vi "Main.vi"(11 "Module Admin":refnum<class "Delacor_lib_QMH_Module Admin.lvclass">) -> ()   [LabVIEW 2020, in "Acquisition.lvlib"]
doc: "This template is based off of the Queued Message Handler design pattern and the Queued Message Handler project template that ships with LabVIEW.\n\nThe main difference is that the queue is private to this module and communication between modules is performed via Broadcast and Request events.\n\nRequest events are wrapped in public API methods and are handled in the Event Handling Loop (EHL) of this VI. Any module can register for Broadcast events sent by this module. The EHL generates messages based on user interface actions.\n\nThe Message Handling Loop (MHL) processes messages generated by the EHL, or by other messages. The messages are string values, so new messages can be added easily to the Message Cases case structure in the MHL. Each message cluster can also provide an optional value for Message Data, which is a variant that can be converted to whatever message-specific data is required.\n_____\nBased on Delacor QMH Project Template 4.0.0.47.\n_____\nBased on DQMH Project Template 6.0.0.91."
uses:
  Acquisition.lvlib
  <vilib>/Delacor/Delacor QMH/Libraries/Module Admin_class/Delacor_lib_QMH_Module Admin.lvclass
  Module Data--cluster.ctl
  Settings Editor/DAQmx Timing--cluster.ctl
  Settings Editor/DAQmx Trigger Settings--cluster.ctl
  Settings Editor/DAQmx Config--cluster.ctl
  Stop Argument--cluster.ctl
  <vilib>/Delacor/Delacor QMH/Libraries/Message Queue_class/Delacor_lib_QMH_Message Queue.lvclass/Delacor_lib_QMH_Message Queue.ctl
  <vilib>/Delacor/Delacor QMH/Libraries/Module Admin_class/Delacor_lib_QMH_Module Admin.lvclass/Delacor_lib_QMH_Module Admin.ctl
  Start Acquiring Argument--cluster.ctl
  Start Acquiring (Reply Payload)--cluster.ctl
  Stop Acquiring Argument--cluster.ctl
  Settings Editor/Update Application Settings (Reply Payload)--cluster.ctl
  Settings Editor/Settings--cluster.ctl
  <vilib>/Utility/miscctls.llb/LVPointTypeDef.ctl
  <vilib>/Delacor/Delacor QMH/Libraries/Message Queue_class/Delacor_lib_QMH_Enqueue Message (Single).vi
  <vilib>/Delacor/Delacor QMH/Libraries/Module Admin_class/Delacor_lib_QMH_Get External Launch.vi
  <vilib>/Utility/error.llb/Error Cluster From Error Code.vi
  <vilib>/ErrorRing/Error Ring.xnode
  <vilib>/Delacor/Delacor QMH/Libraries/Message Queue_class/Delacor_lib_QMH_Message Queue.lvclass
  Settings Editor/Settings Editor.lvlib
  Logger/Logger.lvlib
panel:
  out "Settings":T1={"HW Refnum"="", "DAQmx Timing Settings"={"rate"=0.0, "source"="OnboardClock", "sample mode"=10178, "samples per channel"=1000}, "Trigger Settings"={"Trigger Type"=enum."No Trigger", "Digital Start"={"Source"="", "Digital Start Trigger Edge"=10280}, "Digital Pause"={"Source"="", "Digital Pause Trigger Pause When"=10192}, "Digital Reference"={"Source"="", "Digital Start Trigger Edge"=10280, "Digital Reference Pretrigger Samples"=0}, "Analog Start"={"Source"="", "Analog Slope"=10280, "Analog Start Trigger Hysteresis"=0.0, "Analog Start Trigger Level"=0.0}, "Analog Pause"={"Source"="", "Analog Start Trigger Level"=0.0, "Analog Pause Trigger Pause When"=10093}, "Analog Reference"={"Source"="", "Slope"=10280, "Pretrigger Samples"=0, "Level"=0.0}, "Time Start"={"Select Time\nManually"=FALSE, "When"=timestamp(0 s since 1904-01-01)}}, "DAQmx Config"=[], "Calibration Array"=[{"Slope"=1.0, "Offset"=0.0}]} {"DAQmx Config"."Unit" items=["Volts", "From Custom Scale"]; "Trigger Settings"."Time Start"."When" format="%<%x %.3X>T"; "Trigger Settings"."Analog Reference"."Level" format="%0.2f"; "Trigger Settings"."Analog Reference"."Slope" items=["Rising"=10280, "Falling"=10171]; "Trigger Settings"."Analog Pause"."Analog Pause Trigger Pause When" items=["Above Level"=10093, "Below Level"=10107]; "Trigger Settings"."Analog Pause"."Analog Start Trigger Level" format="%0.2f"; "Trigger Settings"."Analog Start"."Analog Start Trigger Level" format="%0.2f"; "Trigger Settings"."Analog Start"."Analog Start Trigger Hysteresis" format="%.2f"; "Trigger Settings"."Analog Start"."Analog Slope" items=["Rising"=10280, "Falling"=10171]; "Trigger Settings"."Digital Reference"."Digital Start Trigger Edge" items=["Rising"=10280, "Falling"=10171]; "Trigger Settings"."Digital Pause"."Digital Pause Trigger Pause When" items=["High"=10192, "Low"=10214]; "Trigger Settings"."Digital Start"."Digital Start Trigger Edge" items=["Rising"=10280, "Falling"=10171]; "DAQmx Timing Settings"."sample mode" items=["Finite Samples"=10178, "Continuous Samples"=10123, "Hardware Timed Single Point"=12522]; "DAQmx Timing Settings"."rate" format="%0.2f"}
  out "Graph Data":waveform(dbl)[](array[waveform])
  out "error out":errorcluster
  # "This is a headless module. Show its panel to confirm that the Settings are updated correctly and other debugging tasks. Use the Settings Editor to change the settings for this module."
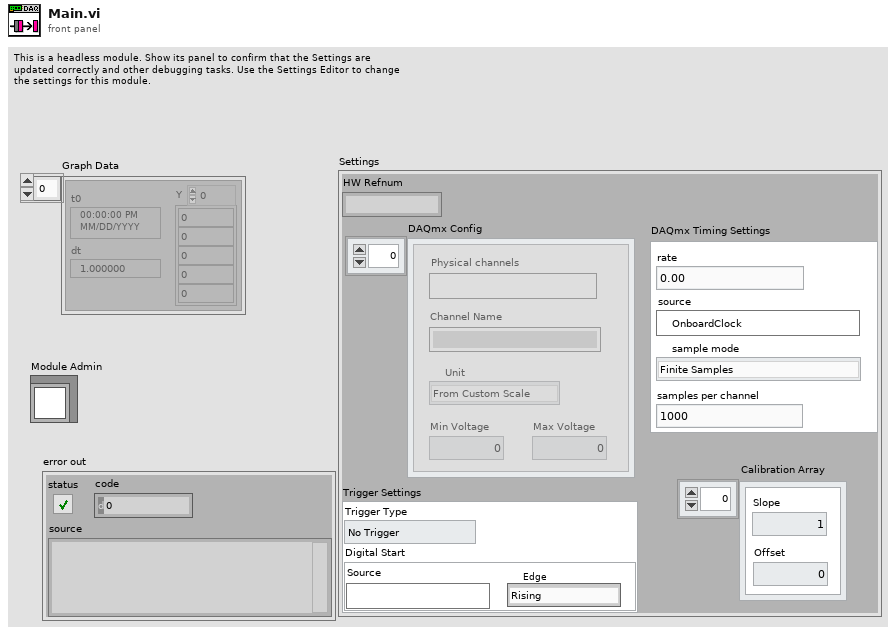
[diagram p1: front panel]
types:
  T1 = typedef "Acquisition.lvlib/Module Data--cluster.ctl" = cluster{"HW Refnum":string, "DAQmx Timing Settings":T2, "Trigger Settings":T3, "DAQmx Config":T4, "Calibration Array":cluster{"Slope":dbl, "Offset":dbl}[]}
  T2 = typedef "Settings Editor.lvlib/DAQmx Timing--cluster.ctl" = cluster{"rate":dbl, "source":tag, "sample mode":i32, "samples per channel":i32}
  T3 = typedef "Settings Editor.lvlib/DAQmx Trigger Settings--cluster.ctl" = cluster{"Trigger Type":enum32{"No Trigger", "Digital Start", "Digital Pause", "Digital Reference", "Analog Start", "Analog Pause", "Analog Reference", "Time Start"}, "Digital Start":cluster{"Source":tag, "Digital Start Trigger Edge":i32}, "Digital Pause":cluster{"Source":tag, "Digital Pause Trigger Pause When":i32}, "Digital Reference":cluster{"Source":tag, "Digital Start Trigger Edge":i32, "Digital Reference Pretrigger Samples":u32}, "Analog Start":cluster{"Source":string, "Analog Slope":i32, "Analog Start Trigger Hysteresis":dbl, "Analog Start Trigger Level":dbl}, "Analog Pause":cluster{"Source":string, "Analog Start Trigger Level":dbl, "Analog Pause Trigger Pause When":i32}, "Analog Reference":cluster{"Source":string, "Slope":i32, "Pretrigger Samples":u32, "Level":dbl}, "Time Start":cluster{"Select Time\nManually":bool, "When":timestamp}}
  T4 = typedef "Settings Editor.lvlib/DAQmx Config--cluster.ctl" = cluster{"Physical channels":tag, "Channel Name":string, "Unit":i32, "Min Voltage":dbl, "Max Voltage":dbl}[]
  T5 = typedef "Settings Editor.lvlib/Broadcast Events--cluster.ctl" = cluster{"Module Did Init":refnum<user-event>, "Status Updated":refnum<user-event>, "Error Reported":refnum<user-event>, "Module Did Stop":refnum<user-event>, "Update Module Execution Status":refnum<user-event>, "Application Settings Updated":refnum<user-event>}
  T6 = typedef "Acquisition.lvlib/Request Events--cluster.ctl" = cluster{"Stop Module":refnum<user-event>, "Show Panel":refnum<user-event>, "Hide Panel":refnum<user-event>, "Get Module Execution Status":refnum<user-event>, "Show Diagram":refnum<user-event>, "Stop Acquiring":refnum<user-event>, "Wakeup Helper Loop":refnum<user-event>, "Change Settings":refnum<user-event>, "Calibrate DAQ":refnum<user-event>, "Start Acquiring":refnum<user-event>}
  T7 = enum32{"invalid lock state", "Not Locked", "Locked (No Password)", "Password-protected"}
  T8 = typedef "Acquisition.lvlib/Stop Argument--cluster.ctl" = cluster{"Origin":string, "Exit via Stop Module Req?":bool, "Wait for Module to stop?":bool}
  T9 = typedef "Acquisition.lvlib/Start Acquiring Argument--cluster.ctl" = cluster{"Wait Notifier":refnum<notifier>, "wait for reply":bool}
  T10 = typedef "Acquisition.lvlib/Stop Acquiring Argument--cluster.ctl" = cluster{"Boolean":bool}
  T11 = typedef "Settings Editor.lvlib/Update Application Settings (Reply Payload)--cluster.ctl" = cluster{"Settings":T12, "Update Settings_error":errorcluster}
  T12 = typedef "Settings Editor.lvlib/Settings--cluster.ctl" = cluster{"Calibration Array":cluster{"Slope":dbl, "Offset":dbl}[], "Hardware Config Cluster":T4, "Trigger Settings":T3, "Log File Base Path":path, "DAQmx Timing Settings":T2}
  T13 = typedef "LVPointTypeDef.ctl" = cluster{"Horizontal":i16, "Vertical":i16}
  T14 = enum32{"Invalid", "Standard", "Closed", "Hidden", "Minimized", "Maximized"}
  T15 = typedef "Acquisition.lvlib/Start Acquiring (Reply Payload)--cluster.ctl" = cluster{"HW ID":string, "Start Acquiring_error":errorcluster}
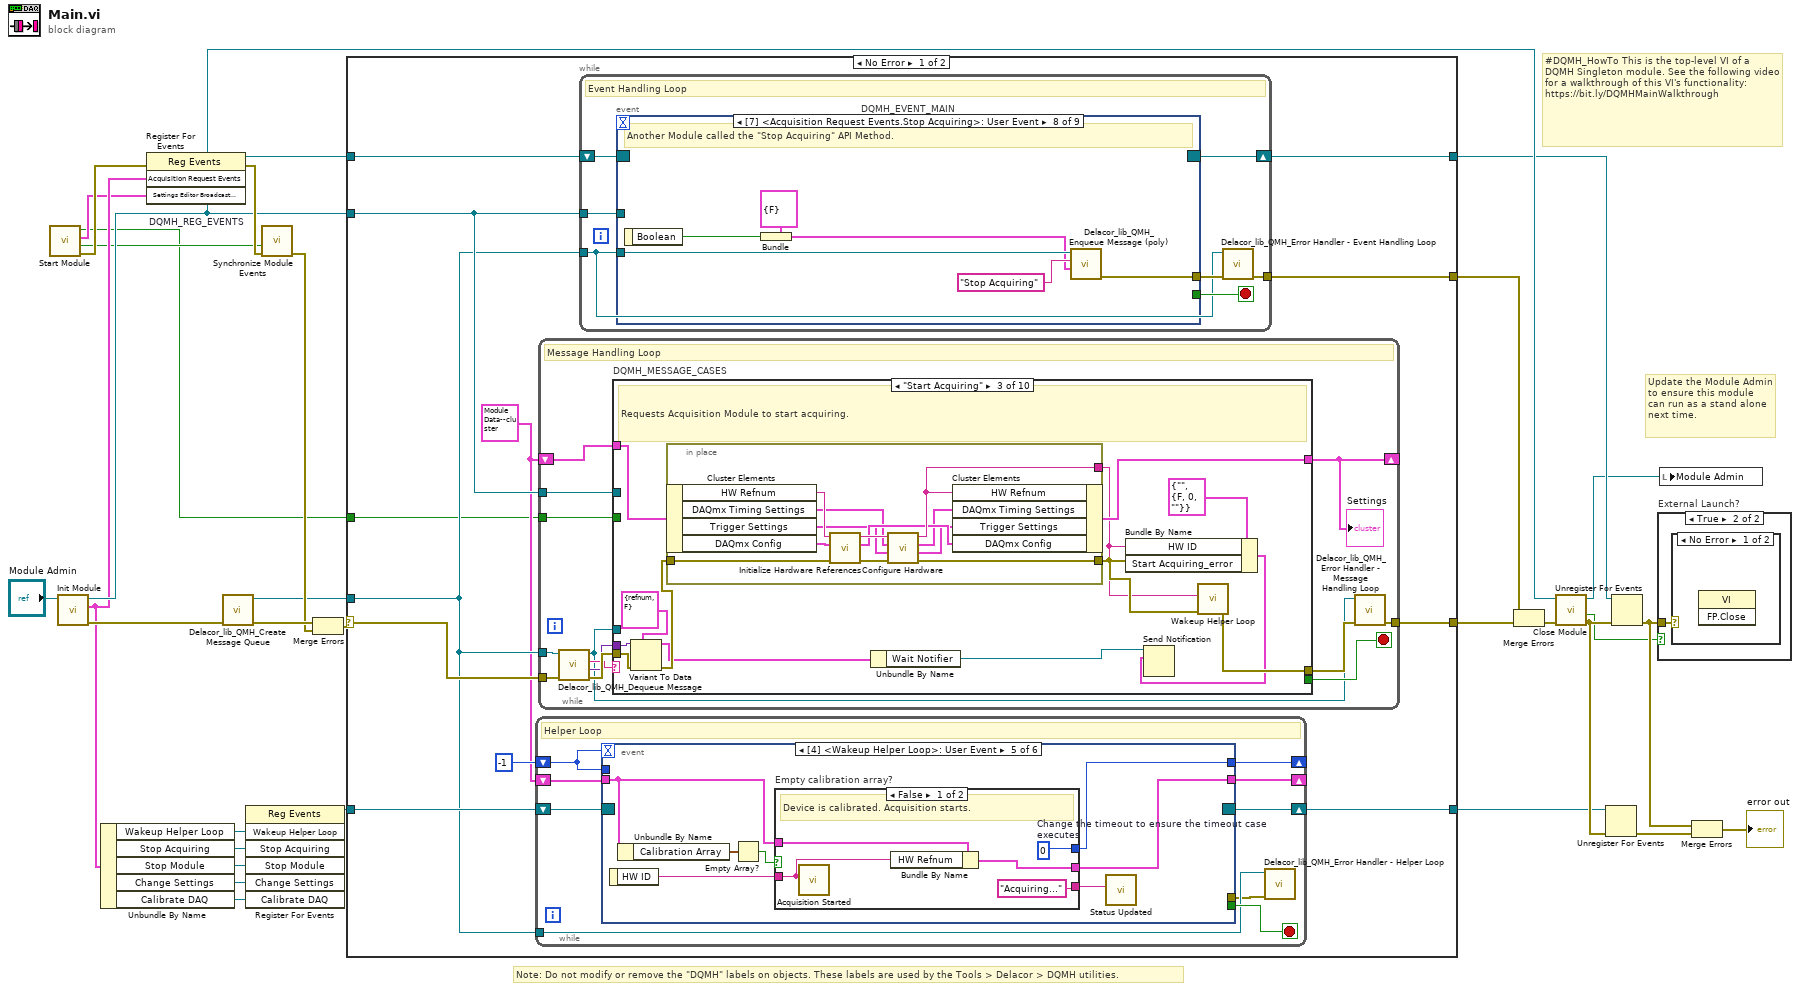
[diagram p0: block diagram]
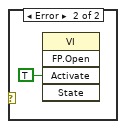
[diagram p3: hidden frame]
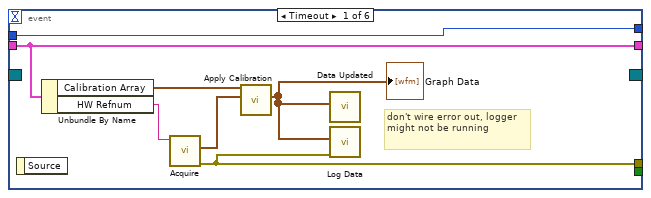
[diagram p4: hidden frame]
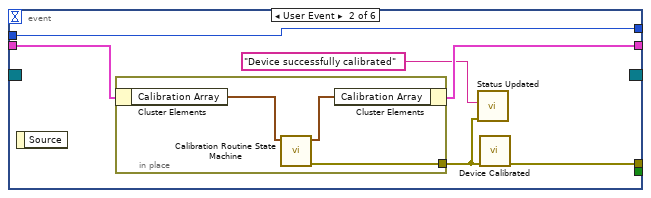
[diagram p5: hidden frame]
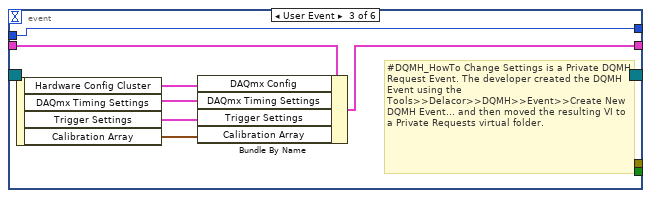
[diagram p6: hidden frame]
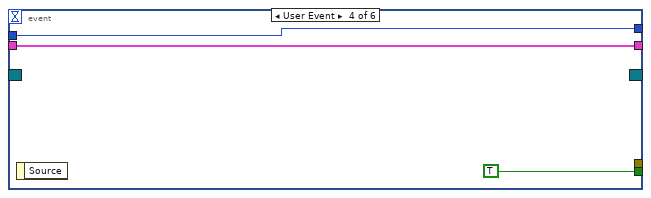
[diagram p7: hidden frame]
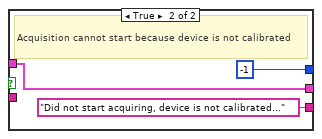
[diagram p8: hidden frame]
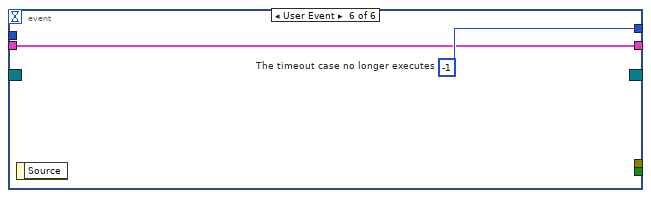
[diagram p9: hidden frame]
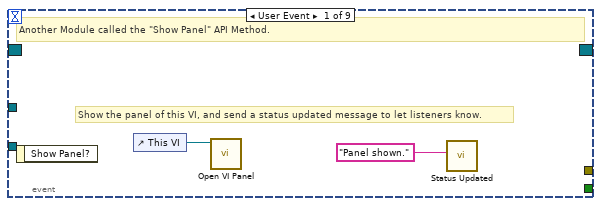
[diagram p10: hidden frame]
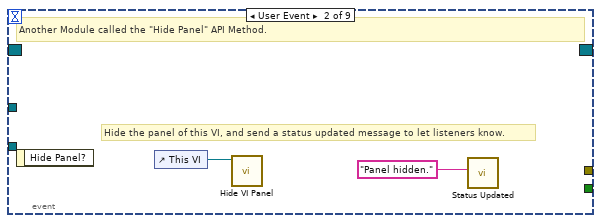
[diagram p11: hidden frame]
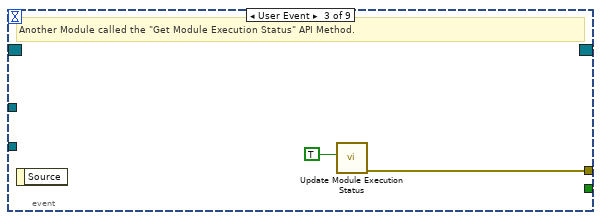
[diagram p12: hidden frame]
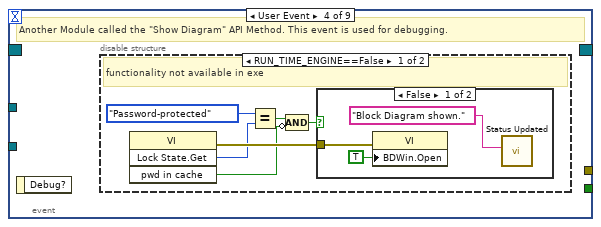
[diagram p13: hidden frame]
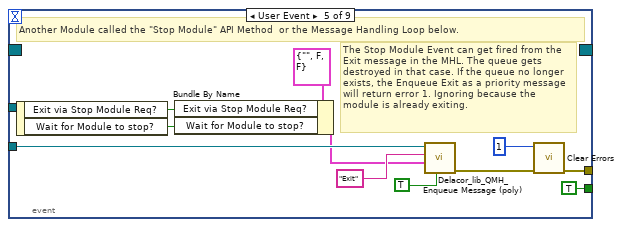
[diagram p16: hidden frame]
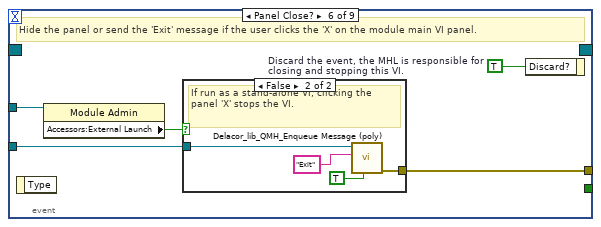
[diagram p17: hidden frame]
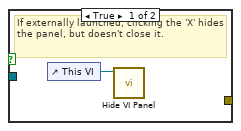
[diagram p18: hidden frame]
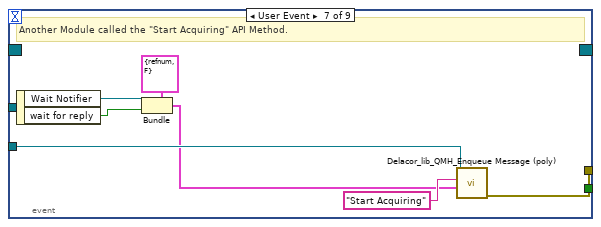
[diagram p19: hidden frame]
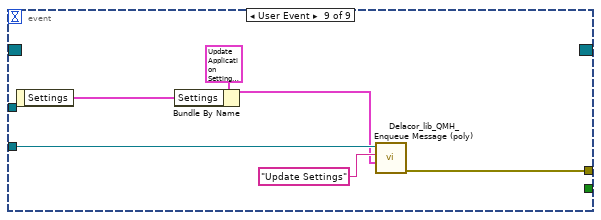
[diagram p20: hidden frame]
diagram:
  # "#DQMH_HowTo This is the top-level VI of a DQMH Singleton module. See the following video for a walkthrough of this VI's functionality: https://bit.ly/DQMHMainWalkthrough"
  # "Note: Do not modify or remove the \"DQMH\" labels on objects. These labels are used by the Tools > Delacor > DQMH utilities."
  # "Update the Module Admin to ensure this module can run as a stand alone next time."
  n1 = call "Start Module.vi"() -> ("error out"=w24:errorcluster, "Wait for Event Sync?"=w5:bool, "Settings Editor Broadcast Events"=w6:T5, "Module Was Already Running?"=w1:bool)  [unwired: 8 in]
  n2 = call "Init Module.vi"("Singleton Module Admin in"="Module Admin") -> ("error out"=w30:errorcluster, "Acquisition Request Events"=w11:T6, "Singleton Module Admin out"=w18:refnum<class "Delacor_lib_QMH_Module Admin.lvclass">)  [unwired: 8 in]
  n3 = Unbundle By Name(w11) -> ("Wakeup Helper Loop"=w7:refnum<user-event>, "Stop Acquiring"=w10:refnum<user-event>, "Stop Module"=w9:refnum<user-event>, "Change Settings"=w4:refnum<user-event>, "Calibrate DAQ"=w3:refnum<user-event>)
  n4 = register-events "DQMH_REG_EVENTS"(error in=w24, w11, w6) -> (reference out=w16:refnum<event-registration>, error out=w23:errorcluster)  [unwired: 1 in]
  n5 = call <vilib>:"Delacor_lib_QMH_Create Message Queue.vi"("error in"=w30) -> ("error out"=w26:errorcluster, "Message Queue"=w15:refnum<class "Delacor_lib_QMH_Message Queue.lvclass">)  [unwired: 9 in]
  n6 = register-events(w7, w10, w9, w4, w3) -> (reference out=w8:refnum<event-registration>)  [unwired: 2 in, 1 out]
  n7 = call "Synchronize Module Events.vi"("error in (no error)"=w23, "Wait for Event Sync?"=w5) -> ("error out"=w22:errorcluster)  [unwired: 9 in]
  n8 = Merge Errors(w26, w22) -> (w25:errorcluster)
  n9 = case shown="No Error" w25 {
    selector: w25 -> [w41 w301]
    tunnel: [w43 w300] -> w31
    tunnel: [w40 w309] -> w17
    tunnel: w16 -> [w39 w309]
    tunnel: w15 -> [w35 w302]
    tunnel: [w42 _] -> w29
    tunnel: w18 -> [w38 w305]
    tunnel: w8 -> [w36 w304]
    tunnel: [w33 w304] -> w2
    tunnel: w1 -> [w32 w303]
    frame No Error {
      w34 = T1 {"HW Refnum"="", "DAQmx Timing Settings"={"rate"=0.0, "source"="OnboardClock", "sample mode"=10178, "samples per channel"=1000}, "Trigger Settings"={"Trigger Type"=enum."No Trigger", "Digital Start"={"Source"="", "Digital Start Trigger Edge"=10280}, "Digital Pause"={"Source"="", "Digital Pause Trigger Pause When"=10192}, "Digital Reference"={"Source"="", "Digital Start Trigger Edge"=10280, "Digital Reference Pretrigger Samples"=0}, "Analog Start"={"Source"="", "Analog Slope"=10280, "Analog Start Trigger Hysteresis"=0.0, "Analog Start Trigger Level"=0.0}, "Analog Pause"={"Source"="", "Analog Start Trigger Level"=0.0, "Analog Pause Trigger Pause When"=10093}, "Analog Reference"={"Source"="", "Slope"=10280, "Pretrigger Samples"=0, "Level"=0.0}, "Time Start"={"Select Time\nManually"=FALSE, "When"=timestamp(0 s since 1904-01-01)}}, "DAQmx Config"=[{"Physical channels"="", "Channel Name"="", "Unit"=1, "Min Voltage"=0.0, "Max Voltage"=0.0}], "Calibration Array"=[{"Slope"=1.0, "Offset"=0.0}]} ("Data Cluster")
      n10 = while {
        shift-right: [w52] -> _
        shift-left: -1 -> [w51]
        tunnel: w35 -> [w45]
        shift-right: [w48] -> _
        shift-left: w34 -> [w47]
        shift-right: [w46] -> w33
        shift-left: w36 -> [w50]
        stop <- w49 stop-if-true
        # "Helper Loop"
        n11 = event shown="[4] <Wakeup Helper Loop>: User Event" {
          selector: w50 -> [_ _ _ _ _ _]
          dyn-events: [_ _ _ _ _ _] -> w46
          timeout: w51 -> [_ _ _ _ _ _]
          tunnel: [w58 w64 w75 w78 w84 w95] -> w52
          tunnel: w51 -> [w58 w64 w75 w78 _ _]
          tunnel: [_ _ _ TRUE _ _] -> w49
          tunnel: [w59 w65 _ _ _ _] -> w44
          tunnel: [w57 w62 w73 w76 w80 w94] -> w48
          tunnel: w47 -> [w57 w63 w74 w76 w79 w94]
          event Timeout {
            # "don't wire error out, logger might not be running"
            n12 = event-data() -> ()  [unwired: 1 in, 1 out]
            n13 = Unbundle By Name(w57) -> ("Calibration Array"=w55:cluster{"Slope":dbl, "Offset":dbl}[], "HW Refnum"=w53:string)
            n14 = call "Acquire.vi"("HW Refnum In"=w53) -> ("error out"=w59:errorcluster, "Graph Data"=w56:waveform(dbl)[])  [unwired: 8 in, 1 out]
            n15 = call "Apply Calibration.vi"("Graph Data"=w56, "Calibration Array"=w55) -> ("Calibrated Data"=w54:waveform(dbl)[])  [unwired: 9 in]
            "Graph Data" <- w54
            n16 = call "Data Updated.vi"("Graph Data"=w54) -> ()  [unwired: 10 in, 1 out]
            n17 = call "Log Data.vi"("error in (no error)"=w59, "Waveforms"=w54) -> ()  [unwired: 9 in, 1 out]
          }
          event User Event {
            n18 = event-data() -> ()  [unwired: 1 in, 1 out]
            n19 = in-place {
              in-place-border: [w68] -> w61
              n20 = in-place-cluster #1(w63) -> ("Calibration Array"=w67:cluster{"Slope":dbl, "Offset":dbl}[])
              n21 = call "Calibration Routine State Machine.vi"("Calibration Array In"=w67) -> ("error out"=w68:errorcluster, "Calibration Array Out"=w66:cluster{"Slope":dbl, "Offset":dbl}[])  [unwired: 9 in]
              n22 = in-place-cluster #1("Calibration Array"=w66) -> (w62:T1)
            }
            n23 = call "Status Updated.vi"("error in (no error)"=w61, "Status"="Device successfully calibrated") -> ()  [unwired: 9 in, 1 out]
            n24 = call "Device Calibrated.vi"("error in (no error)"=w61) -> ("error out"=w65:errorcluster)  [unwired: 10 in]
          }
          event User Event {
            # "#DQMH_HowTo Change Settings is a Private DQMH Request Event. The developer created the DQMH Event using the Tools>>Delacor>>DQMH>>Event>>Create New DQMH Event... and then moved the resulting VI to a Private Requests virtual folder."
            n25 = event-data() -> ("Hardware Config Cluster"=w72:T4, "DAQmx Timing Settings"=w71:T2, "Trigger Settings"=w70:T3, "Calibration Array"=w69:cluster{"Slope":dbl, "Offset":dbl}[])  [unwired: 1 in]
            n26 = Bundle By Name(cluster=w74, "DAQmx Config"=w72, "DAQmx Timing Settings"=w71, "Trigger Settings"=w70, "Calibration Array"=w69) -> (w73:T1)
          }
          event User Event {
            n27 = event-data() -> ()  [unwired: 1 in, 1 out]
          }
          event User Event {
            n28 = event-data() -> ("HW ID"=w82:string)  [unwired: 1 in]
            n29 = Unbundle By Name(w79) -> ("Calibration Array"=w81:cluster{"Slope":dbl, "Offset":dbl}[])
            n30 = Empty Array?(array=w81) -> (empty?=w85:bool)
            n31 = case "Empty calibration array?" shown="False" w85 {
              tunnel: ["Acquiring..." ("Status") "Did not start acquiring, device is not calibrated..." ("Status")] -> w83
              tunnel: [w90 -1] -> w84
              tunnel: w82 -> [w87 _]
              tunnel: w79 -> [w88 w91]
              tunnel: [w86 w91] -> w80
              frame False {
                w90 = 0  # Change the timeout to ensure the timeout case executes
                # "Device is calibrated. Acquisition starts."
                n32 = call "Acquisition Started.vi"("HW ID"=w87) -> ()  [unwired: 10 in, 1 out]
                n33 = Bundle By Name(cluster=w88, "HW Refnum"=w87) -> (w86:T1)
              }
              frame True {
                # "Acquisition cannot start because device is not calibrated"
              }
            }
            n34 = call "Status Updated.vi"("Status"=w83) -> ()  [unwired: 10 in, 1 out]
          }
          event User Event {
            w95 = -1  # The timeout case no longer executes
            n35 = event-data() -> ()  [unwired: 1 in, 1 out]
          }
        }
        n36 = call-dynamic "Delacor_lib_QMH_Error Handler - Helper Loop.vi"("error in"=w44, "Message Queue in"=w45) -> ()  [unwired: 8 in, 2 out]
      }
      n37 = while {
        tunnel: w35 -> [w161]
        shift-right: [w165] -> _
        shift-left: w34 -> [w166]
        tunnel: w41 -> [w169]
        tunnel: [w167] -> w43
        tunnel: w38 -> [w159]
        tunnel: w32 -> [w158]
        stop <- w164 stop-if-true
        # "Message Handling Loop"
        n38 = call-dynamic "Delacor_lib_QMH_Dequeue Message.vi"("error in"=w169, "Message Queue in"=w161) -> ("error out"=w168:errorcluster, "Message Data"=w162:variant, "Message"=w163:string, "Message Queue out"=w160:refnum<class "Delacor_lib_QMH_Message Queue.lvclass">)  [unwired: 6 in]
        n39 = case "DQMH_MESSAGE_CASES" shown="\"Start Acquiring\"" w163 {
          selector: w163 -> [_ _ _ _ _ _ _ _ _ w287]
          tunnel: w160 -> [_ _ _ _ _ _ _ w252 w276 _]
          tunnel: w168 -> [w195 w199 w212 w232 w244 w247 w249 w259 w283 w290]
          tunnel: [w192 w199 w210 w230 w238 w246 w249 w255 w280 w291] -> w170
          tunnel: w166 -> [w182 w198 w200 w227 w241 w245 w248 w254 w268 w288]
          tunnel: [w177 w198 w208 w227 w241 w245 w248 w254 w268 w288] -> w165
          tunnel: [_ _ _ _ _ _ _ _ w275 _] -> w164
          tunnel: w162 -> [_ _ w207 w229 w242 _ _ w253 w274 _]
          tunnel: w159 -> [w183 _ _ _ _ _ _ w251 w269 _]
          tunnel: w158 -> [_ _ _ _ _ _ _ _ w266 _]
          frame "Initialize" {
            # "Initialize - Any operation that needs to be done before the module can receive messages. Synchronize Caller Events.vi will inform Start Module.vi that the module has launched and is ready to receive messages. Module Did Init.vi will broadcast that the module initialized."
            n40 = call "Synchronize Caller Events.vi"("error in (no error)"=w195, "Singleton Module Admin in"=w183) -> ("error out"=w194:errorcluster, "Singleton Module Admin out"=w179:refnum<class "Delacor_lib_QMH_Module Admin.lvclass">)  [unwired: 8 in]
            n41 = call "Update Application Settings.vi"("wait for reply (T)"=TRUE) -> ("error out"=w191:errorcluster, "Reply Payload"=w176:T11)  [unwired: 8 in, 1 out]
            n42 = Unbundle By Name(w176) -> ("Settings.Hardware Config Cluster"=w174:T4, "Settings.DAQmx Timing Settings"=w173:T2, "Settings.Trigger Settings"=w172:T3, "Settings.Calibration Array"=w171:cluster{"Slope":dbl, "Offset":dbl}[])
            n43 = property class="Module Admin"(reference=w179) -> ("Accessors:External Launch"=w187:bool)  [unwired: 1 in, 2 out]
            n44 = Select(t=T14."Hidden" ("State"), s=w187, f=T14."Standard" ("State")) -> (s? t:f=w184:T14)
            n45 = Bundle By Name(cluster=w182, "DAQmx Config"=w174, "DAQmx Timing Settings"=w173, "Trigger Settings"=w172, "Calibration Array"=w171) -> (w177:T1)
            n46 = call "Module Name--constant.vi"() -> ("Module Name"=w190:string)  [unwired: 11 in]
            n47 = property class="VI"("Front Panel.Title"=w190) -> (reference out=w189:refnum<vi>, error out=w197:errorcluster)  [unwired: 2 in]
            n48 = call "Module Name--constant.vi"() -> ("Module Name"=w180:string)  [unwired: 11 in]
            n49 = invoke class="VI" method="FP.Open"(reference=w189, error in=w197, "State"=w184) -> (reference out=w188:refnum<vi>, error out=w196:errorcluster)  [unwired: 2 in, 3 out]
            n50 = call "Module Did Init.vi"("error in (no error)"=w194, "Initialized?"=TRUE, "Origin"=w180) -> ("error out"=w193:errorcluster)  [unwired: 8 in]
            n51 = invoke class="VI" method="FP.Center"(reference=w188, error in=w196) -> ()  [unwired: 1 in, 3 out]
            n52 = Merge Errors(w193, w191) -> (w192:errorcluster)
            n53 = property on="Pane" class="Pane"("Origin"=T13 {"Horizontal"=0, "Vertical"=0}) -> ()  [unwired: 2 in, 2 out]
          }
          frame "---Module Specific---" {
            # "Separator -- The following cases handle messages specific to this Module."
          }
          frame "Start Acquiring" {
            # "Requests Acquisition Module to start acquiring."
            n54 = Variant To Data(error in=w212, type=T9 {"Wait Notifier"=refnum, "wait for reply"=FALSE} ("Start Acquisition Argument"), Variant=w207) -> (data=w205:T9, error out=w209:errorcluster)
            n55 = in-place {
              in-place-border: [w224] -> w211
              in-place-border: w209 -> [w223]
              in-place-border: [w220] -> w201
              n56 = in-place-cluster #2(w200) -> ("HW Refnum"=w221:string, "DAQmx Timing Settings"=w216:T2, "Trigger Settings"=w215:T3, "DAQmx Config"=w218:T4)
              n57 = call "Initialize Hardware References.vi"("error in (no error)"=w223, "Hardware Config \nCluster"=w218, "HW Refnum"=w221) -> ("error out"=w222:errorcluster, "Hardware Config Out"=w217:T4, "HW Refnum"=w219:string)  [unwired: 6 in]
              n58 = call "Configure Hardware.vi"("error in (no error)"=w222, "Trigger Settings"=w215, "DAQmx Timing Settings In"=w216, "HW Refnum In"=w219) -> ("error out"=w224:errorcluster, "Trigger Settings Out"=w213:T3, "DAQmx Timing Settings Out"=w214:T2, "HW Refnum Out"=w220:string)  [unwired: 4 in]
              n59 = in-place-cluster #2("HW Refnum"=w220, "DAQmx Timing Settings"=w214, "Trigger Settings"=w213, "DAQmx Config"=w217) -> (w208:T1)
            }
            n60 = Unbundle By Name(w205) -> ("Wait Notifier"=w204:refnum<notifier>)
            n61 = Bundle By Name(cluster=T15 {"HW ID"="", "Start Acquiring_error"={"status"=FALSE, "code"=0, "source"=""}} ("Start Acquisition (Reply Payload)"), "HW ID"=w201, "Start Acquiring_error"=w211) -> (w203:T15)
            n62 = Send Notification(notification=w203, notifier=w204) -> ()  [unwired: 1 in, 2 out]
            n63 = call "Wakeup Helper Loop.vi"("error in (no error)"=w211, "HW ID"=w201) -> ("error out"=w210:errorcluster)  [unwired: 9 in]
          }
          frame "Stop Acquiring" {
            # "Requests the Acquisition Module to stop acquiring"
            n64 = Variant To Data(error in=w232, type=T10 {"Boolean"=FALSE} ("Stop Acquiring Argument"), Variant=w229) -> (error out=w231:errorcluster)  [unwired: 1 out]
            n65 = Unbundle By Name(w227) -> ("HW Refnum"=w226:string)
            n66 = call "Stop Acquisition.vi"("error in (no error)"=w231, "HW Refnum In"=w226) -> ("error out"=w230:errorcluster)  [unwired: 9 in]
            n67 = call "Acquisition Stopped.vi"("error in (no error)"=w230) -> ()  [unwired: 10 in, 1 out]
            n68 = call "Status Updated.vi"("error in (no error)"=w230, "Status"="Acquisition Stopped") -> ()  [unwired: 9 in, 1 out]
          }
          frame "Update Settings" {
            # "Send the Change Settings event to the helper loop."
            # "The Settings Editor broadcasted that the settings have changed."
            n69 = Variant To Data(error in=w244, type=T11 {"Settings"={"Calibration Array"=[], "Hardware Config Cluster"=[{"Physical channels"="", "Channel Name"="", "Unit"=1, "Min Voltage"=0.0, "Max Voltage"=0.0}], "Trigger Settings"={"Trigger Type"=enum."No Trigger", "Digital Start"={"Source"="", "Digital Start Trigger Edge"=10280}, "Digital Pause"={"Source"="APFI0", "Digital Pause Trigger Pause When"=10192}, "Digital Reference"={"Source"="", "Digital Start Trigger Edge"=10280, "Digital Reference Pretrigger Samples"=0}, "Analog Start"={"Source"="", "Analog Slope"=10093, "Analog Start Trigger Hysteresis"=0.0, "Analog Start Trigger Level"=0.0}, "Analog Pause"={"Source"="", "Analog Start Trigger Level"=0.0, "Analog Pause Trigger Pause When"=10093}, "Analog Reference"={"Source"="", "Slope"=10280, "Pretrigger Samples"=0, "Level"=0.0}, "Time Start"={"Select Time\nManually"=FALSE, "When"=timestamp(0 s since 1904-01-01)}}, "Log File Base Path"=path "", "DAQmx Timing Settings"={"rate"=1000.0, "source"="OnboardClock", "sample mode"=10178, "samples per channel"=1000}}, "Update Settings_error"={"status"=FALSE, "code"=0, "source"=""}} ("Settings Updated Argument"), Variant=w242) -> (data=w239:T11, error out=w243:errorcluster)
            n70 = Unbundle By Name(w239) -> ("Settings.Hardware Config Cluster"=w236:T4, "Settings.DAQmx Timing Settings"=w235:T2, "Settings.Trigger Settings"=w233:T3, "Settings.Calibration Array"=w234:cluster{"Slope":dbl, "Offset":dbl}[])
            n71 = call "Change Settings.vi"("DAQmx Config"=w236, "DAQmx Timing Settings"=w235, "Trigger Settings"=w233, "Calibration Array"=w234, "error in (no error)"=w243) -> ("error out"=w238:errorcluster)  [unwired: 10 in]
            n72 = call "Status Updated.vi"("error in (no error)"=w238, "Status"="Settings Updated") -> ()  [unwired: 9 in, 1 out]
          }
          frame "---Copy This Frame---" {
            # "Duplicate this frame when creating new messages.  Change this comment in the duplicated frame to describe this message."
            n73 = Merge Errors(w247) -> (w246:errorcluster)
          }
          frame "---Exit and Error Handling---" {
            # "Separator - The following cases handle errors and exit messages."
          }
          frame "Error" {
            # "Error - Check the error message data and respond accordingly. This message is sent by the \"Error Handler\" VIs at the end of each loop in this application."
            n74 = Variant To Data(error in=w259, type=errorcluster {"status"=FALSE, "code"=0, "source"=""} ("error constant"), Variant=w253) -> (data=w260:errorcluster, error out=w257:errorcluster)
            n75 = property class="Module Admin"(reference=w251) -> ("Accessors:External Launch"=w250:bool)  [unwired: 1 in, 2 out]
            n76 = call "Error Reported.vi"("Error"=w260) -> ()  [unwired: 10 in, 1 out]
            n77 = case shown="True" w250 {
              tunnel: [w265 _] -> w256
              tunnel: w252 -> [w263 _]
              tunnel: w260 -> [w264 _]
              frame False {
                # "If the module is running standalone, then pop up an error dialog and call the \"Exit\" message."
                n78 = call <vilib>:"Simple Error Handler.vi"("error in (no error)"=w264) -> ()  [unwired: 4 in, 5 out]
                n79 = call-poly <vilib>:"Delacor_lib_QMH_Enqueue Message (poly).vi"("Priority Message? (F)"=TRUE, "Message"="Exit", "Message Queue in"=w263) -> ("error out"=w265:errorcluster)  [unwired: 7 in, 1 out]
              }
              frame True {
                # "If the module was launched externally, calling the Error Reported broadcast VI is the only action performed by the \"Error\" message. The module's caller can then process the error appropriately."
              }
            }
            n80 = Merge Errors(w257, w256) -> (w255:errorcluster)
            n81 = local write "error out"(w255) -> ()
          }
          frame "Exit" {
            w273 = 91  # 91: not all Exit messages will have an argument
            w275 = TRUE  # Stop the VI
            # "Release the message queue reference"
            # "Exit - Exit the application."
            n82 = Variant To Data(error in=w283, type=T8 {"Origin"="", "Exit via Stop Module Req?"=FALSE, "Wait for Module to stop?"=FALSE} ("Stop Argument"), Variant=w274) -> (data=w271:T8, error out=w279:errorcluster)
            n83 = call <vilib>:"Clear Errors.vi"("error in (no error)"=w279, "specific error code to clear (0: all)"=w273) -> ("error out"=w282:errorcluster)  [unwired: 4 in, 1 out]
            n84 = Unbundle By Name(w268) -> ("HW Refnum"=w267:string)
            n85 = control-ref of="This VI"() -> (w270:refnum<vi>)
            n86 = call "Handle Exit.vi"("Stop Argument"=w271, "Admin in"=w269, "VI reference"=w270) -> ("error out"=w278:errorcluster)  [unwired: 7 in, 1 out]
            n87 = call "Close Hardware References.vi"("HW Refnum in"=w267) -> ("error out"=w277:errorcluster)  [unwired: 9 in, 1 out]
            n88 = call-dynamic "Delacor_lib_QMH_Release Message Queue.vi"("error in"=w282, "Message Queue"=w276) -> ("error out"=w281:errorcluster)  [unwired: 9 in]
            n89 = case "Settings Editor was\nalready running?" shown="False" w266 {
              frame False {
                n90 = call "Module Name--constant.vi"() -> ("Module Name"=w285:string)  [unwired: 11 in]
                n91 = call "Stop Module.vi"("Wait for Module to Stop? (F)"=TRUE, "Origin"=w285) -> ()  [unwired: 9 in, 1 out]
              }
              frame True {
                # "Another Module is\nin charge of stopping Settings Editor"
              }
            }
            n92 = Merge Errors(w281, w278, w277) -> (w280:errorcluster)
          }
          frame Default {
            # "'Default' case only runs if there is a message that isn't defined in any of the other cases.  Output a programming error."
            n93 = call "Module Name--constant.vi"() -> ("Module Name"=w286:string)  [unwired: 11 in]
            n94 = xnode "Error Ring"("parameter 0"=w287, "parameter 1"=w286) -> ("error out"=w289:errorcluster)
            n95 = Merge Errors(w290, w289) -> (w291:errorcluster)
          }
        }
        "Settings" <- w165
        n96 = call-dynamic "Delacor_lib_QMH_Error Handler - Message Handling Loop.vi"("error in"=w170, "Message Queue in"=w160) -> ("dup error in"=w167:errorcluster)  [unwired: 8 in, 1 out]
      }
      n97 = while {
        tunnel: w35 -> [w96]
        shift-right: [w99] -> w40
        shift-left: w39 -> [w100]
        tunnel: [w101] -> w42
        tunnel: w38 -> [w97]
        stop <- w98 stop-if-true
        # "Event Handling Loop"
        n98 = event "DQMH_EVENT_MAIN" shown="[7] <Acquisition Request Events.Stop Acquiring>: User Event" {
          selector: w100 -> [_ _ _ _ _ _ _ _ _]
          dyn-events: [_ _ _ _ _ _ _ _ _] -> w99
          timeout: _ -> [_ _ _ _ _ _ _ _ _]
          tunnel: [_ _ _ _ TRUE ("Discard?") _ _ _ _] -> w98
          tunnel: w96 -> [_ _ _ _ w124 w131 w145 w150 w155]
          tunnel: [_ _ w108 _ w127 w133 w141 w151 w157] -> w102
          tunnel: w97 -> [_ _ _ _ _ w130 _ _ _]
          event User Event {
            # "Show the panel of this VI, and send a status updated message to let listeners know."
            # "Another Module called the \"Show Panel\" API Method."
            n99 = event-data() -> ()  [unwired: 1 in, 1 out]
            n100 = control-ref of="This VI"() -> (w104:refnum<vi>)
            n101 = call "Open VI Panel.vi"("VI"=w104) -> ()  [unwired: 10 in, 1 out]
            n102 = call "Status Updated.vi"("Status"="Panel shown." ("format string")) -> ()  [unwired: 10 in, 1 out]
          }
          event User Event {
            # "Hide the panel of this VI, and send a status updated message to let listeners know."
            # "Another Module called the \"Hide Panel\" API Method."
            n103 = event-data() -> ()  [unwired: 1 in, 1 out]
            n104 = control-ref of="This VI"() -> (w106:refnum<vi>)
            n105 = call "Hide VI Panel.vi"("VI"=w106) -> ()  [unwired: 10 in, 1 out]
            n106 = call "Status Updated.vi"("Status"="Panel hidden." ("format string")) -> ()  [unwired: 10 in, 1 out]
          }
          event User Event {
            # "Another Module called the \"Get Module Execution Status\" API Method."
            n107 = event-data() -> ()  [unwired: 1 in, 1 out]
            n108 = call "Update Module Execution Status.vi"("Running?"=TRUE) -> ("error out"=w108:errorcluster)  [unwired: 10 in]
          }
          event User Event {
            # "Another Module called the \"Show Diagram\" API Method. This event is used for debugging."
            n109 = event-data() -> ()  [unwired: 1 in, 1 out]
            n110 = disable-structure shown="RUN_TIME_ENGINE==False" {
              frame condition #0 (active) {
                # "functionality not available in exe"
                n111 = invoke class="VI" method="Lock State.Get"() -> (error out=w114:errorcluster, "Get Lock State"=w113:T7, "pwd in cache"=w110:bool)  [unwired: 4 in, 1 out]
                n112 = Equal?(x=T7."Password-protected", y=w113) -> (x = y?=w111:bool)
                n113 = Compound Arithmetic op=AND(w111, invert w110) -> (w109:bool)
                n114 = case shown="False" w109 {
                  tunnel: w114 -> [w117 _]
                  frame False {
                    n115 = property class="VI"(error in=w117, "BDWin.Open"=TRUE ("Block Diagram Window:Open")) -> ()  [unwired: 1 in, 2 out]
                    n116 = call "Status Updated.vi"("Status"="Block Diagram shown." ("format string")) -> ()  [unwired: 10 in, 1 out]
                  }
                  frame True {
                    # "Password-protected VI, and the password is not in the cache. Do not show the diagram."
                  }
                }
              }
              frame condition #1 {
              }
            }
          }
          event User Event {
            # "The Stop Module Event can get fired from the Exit message in the MHL. The queue gets destroyed in that case. If the queue no longer exists, the Enqueue Exit as a priority message will return error 1. Ignoring because the module is already exiting."
            # "Another Module called the \"Stop Module\" API Method  or the Message Handling Loop below."
            n117 = event-data() -> ("Exit via Stop Module Req?"=w120:bool, "Wait for Module to stop?"=w119:bool)  [unwired: 1 in]
            n118 = Bundle By Name(cluster=T8 {"Origin"="", "Exit via Stop Module Req?"=FALSE, "Wait for Module to stop?"=FALSE} ("Stop Argument"), "Exit via Stop Module Req?"=w120, "Wait for Module to stop?"=w119) -> (w118:T8)
            n119 = call-poly <vilib>:"Delacor_lib_QMH_Enqueue Message (poly).vi"("Priority Message? (F)"=TRUE, "Message Data"=w118, "Message"="Exit", "Message Queue in"=w124) -> ("error out"=w128:errorcluster)  [unwired: 6 in, 1 out]
            n120 = call <vilib>:"Clear Errors.vi"("error in (no error)"=w128, "specific error code to clear (0: all)"=1) -> ("error out"=w127:errorcluster)  [unwired: 4 in, 1 out]
          }
          event Panel Close? {
            w132 = TRUE  # Discard the event, the MHL is responsible for closing and stopping this VI.
            # "Hide the panel or send the 'Exit' message if the user clicks the 'X' on the module main VI panel."
            n121 = event-data() -> ()  [unwired: 1 in, 1 out]
            n122 = property class="Module Admin"(reference=w130) -> ("Accessors:External Launch"=w129:bool)  [unwired: 1 in, 2 out]
            n123 = case shown="False" w129 {
              tunnel: w131 -> [_ w137]
              tunnel: [_ w138] -> w133
              frame True {
                # "If externally launched, clicking the 'X' hides the panel, but doesn't close it."
                n124 = control-ref of="This VI"() -> (w134:refnum<vi>)
                n125 = call "Hide VI Panel.vi"("VI"=w134) -> ()  [unwired: 10 in, 1 out]
              }
              frame False {
                # "If run as a stand-alone VI, clicking the panel 'X' stops the VI."
                n126 = call-poly <vilib>:"Delacor_lib_QMH_Enqueue Message (poly).vi"("Priority Message? (F)"=TRUE, "Message"="Exit", "Message Queue in"=w137) -> ("error out"=w138:errorcluster)  [unwired: 7 in, 1 out]
              }
            }
            n127 = event-data("Discard?"=w132) -> ()  [unwired: 1 in, 1 out]
          }
          event User Event {
            # "Another Module called the \"Start Acquiring\" API Method."
            n128 = event-data() -> ("Wait Notifier"=w140:refnum<notifier>, "wait for reply"=w139:bool)  [unwired: 1 in]
            n129 = Bundle(cluster=T9 {"Wait Notifier"=refnum, "wait for reply"=FALSE} ("Start Acquisition Argument"), "Wait Notifier"=w140, "wait for reply"=w139) -> (w142:T9)
            n130 = call-poly <vilib>:"Delacor_lib_QMH_Enqueue Message (poly).vi"("Message Data"=w142, "Message"="Start Acquiring", "Message Queue in"=w145) -> ("error out"=w141:errorcluster)  [unwired: 7 in, 1 out]
          }
          event User Event {
            # "Another Module called the \"Stop Acquiring\" API Method."
            n131 = event-data() -> ("Boolean"=w146:bool)  [unwired: 1 in]
            n132 = Bundle(cluster=T10 {"Boolean"=FALSE} ("Stop Acquiring Argument"), "Boolean"=w146) -> (w147:T10)
            n133 = call-poly <vilib>:"Delacor_lib_QMH_Enqueue Message (poly).vi"("Message Data"=w147, "Message"="Stop Acquiring", "Message Queue in"=w150) -> ("error out"=w151:errorcluster)  [unwired: 7 in, 1 out]
          }
          event User Event {
            n134 = event-data() -> ("Settings"=w152:T12)  [unwired: 1 in]
            n135 = Bundle By Name(cluster=T11 {"Settings"={"Calibration Array"=[], "Hardware Config Cluster"=[{"Physical channels"="", "Channel Name"="", "Unit"=1, "Min Voltage"=0.0, "Max Voltage"=0.0}], "Trigger Settings"={"Trigger Type"=enum."No Trigger", "Digital Start"={"Source"="", "Digital Start Trigger Edge"=10280}, "Digital Pause"={"Source"="APFI0", "Digital Pause Trigger Pause When"=10192}, "Digital Reference"={"Source"="", "Digital Start Trigger Edge"=10280, "Digital Reference Pretrigger Samples"=0}, "Analog Start"={"Source"="", "Analog Slope"=10093, "Analog Start Trigger Hysteresis"=0.0, "Analog Start Trigger Level"=0.0}, "Analog Pause"={"Source"="", "Analog Start Trigger Level"=0.0, "Analog Pause Trigger Pause When"=10093}, "Analog Reference"={"Source"="", "Slope"=10280, "Pretrigger Samples"=0, "Level"=0.0}, "Time Start"={"Select Time\nManually"=FALSE, "When"=timestamp(0 s since 1904-01-01)}}, "Log File Base Path"=path "", "DAQmx Timing Settings"={"rate"=1000.0, "source"="OnboardClock", "sample mode"=10178, "samples per channel"=1000}}, "Update Settings_error"={"status"=FALSE, "code"=0, "source"=""}} ("Settings Updated Argument"), "Settings"=w152) -> (w154:T11)
            n136 = call-poly <vilib>:"Delacor_lib_QMH_Enqueue Message (poly).vi"("Message Data"=w154, "Message"="Update Settings", "Message Queue in"=w155) -> ("error out"=w157:errorcluster)  [unwired: 7 in, 1 out]
          }
        }
        n137 = call-dynamic "Delacor_lib_QMH_Error Handler - Event Handling Loop.vi"("error in"=w102, "Message Queue in"=w96) -> ("dup error in"=w101:errorcluster)  [unwired: 8 in, 1 out]
      }
    }
    frame Error {
      # "Synchronize Caller Events.vi will inform Start Module.vi that the module has launched and will let the code calling Start Module.vi register for broadcasts and would permit the caller receive the broadcast that an error occurred at launch time."
      n138 = call "Synchronize Caller Events.vi"("Singleton Module Admin in"=w305) -> ("error out"=w310:errorcluster)  [unwired: 9 in, 1 out]
      n139 = call-dynamic "Delacor_lib_QMH_Release Message Queue.vi"("error in"=w301, "Message Queue"=w302) -> ("error out"=w300:errorcluster)  [unwired: 9 in]
      n140 = call "Module Name--constant.vi"() -> ("Module Name"=w308:string)  [unwired: 11 in]
      n141 = case "Settings Editor was\nalready running?" shown="False" w303 {
        frame False {
          n142 = call "Module Name--constant.vi"() -> ("Module Name"=w313:string)  [unwired: 11 in]
          n143 = call "Stop Module.vi"("Wait for Module to Stop? (F)"=TRUE, "Origin"=w313) -> ()  [unwired: 9 in, 1 out]
        }
        frame True {
          # "Another Module is\nin charge of stopping Settings Editor"
        }
      }
      n144 = Format Into String(format string="An error occurred during initialization. %s is no longer running.", w308) -> (resulting string=w306:string)  [unwired: 2 in, 1 out]
      n145 = Merge Errors(w300, w310) -> (w311:errorcluster)
      n146 = call "Error Reported.vi"("Additional Information"=w306, "Error"=w311) -> ()  [unwired: 9 in, 1 out]
    }
  }
  n147 = Merge Errors(w29, w31) -> (w28:errorcluster)
  n148 = call "Close Module.vi"("error in (no error)"=w28, "Module Admin in"=w18) -> ("error out"=w21:errorcluster, "External Launch"=w12:bool, "Module Admin out"=w13:refnum<class "Delacor_lib_QMH_Module Admin.lvclass">)  [unwired: 7 in]
  n149 = Unregister For Events(event registration refnum=w2, error in=w21) -> (error out=w19:errorcluster)
  n150 = Unregister For Events(event registration refnum=w17, error in=w21) -> (error out=w27:errorcluster)
  n151 = case "External Launch?" shown="True" w12 {
    tunnel: w27 -> [_ w314]
    frame False {
    }
    frame True {
      n152 = case shown="No Error" w314 {
        frame No Error {
          n153 = invoke class="VI" method="FP.Close"() -> ()  [unwired: 3 in, 3 out]
        }
        frame Error {
          n154 = invoke class="VI" method="FP.Open"("Activate"=TRUE ("Activate?")) -> ()  [unwired: 4 in, 5 out]
        }
      }
    }
  }
  n155 = local write "Module Admin"(w13) -> ()
  n156 = Merge Errors(w27, w19) -> (→"error out":errorcluster)
